vi "RSZVB Set Soft Key Label.vi"(8 "error in (no error)":errorcluster {"code" format="%.0x"}, 9 "Label":string, 10 "Key Number (1)":i32=1, 11 "VISA session":refnum<visa-resource-name>) -> (0 "error out":errorcluster {"code" format="%.0x"}, 3 "dup VISA session":refnum<visa-resource-name>)   [LabVIEW 2011]
doc: "This VI assigns the label to the soft key 1...8. The label may contain the '\\n'- character to form multiline labels.\n\nRemote-control command(s):\n:SYSTem:USER:FKEY 0\n:SYSTem:USER:FKEY <1...8>,'<Label>'"
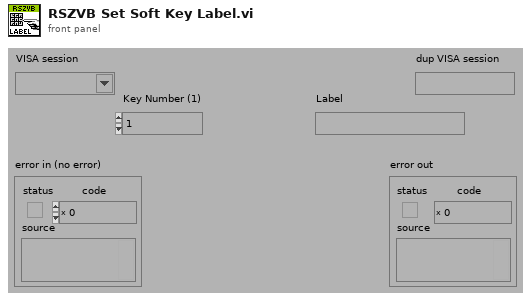
[diagram p1: front panel]
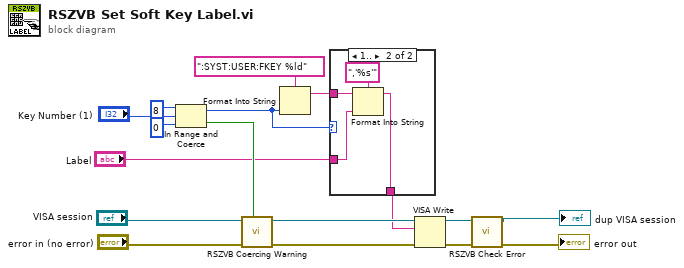
[diagram p0: block diagram]
diagram:
  n1 = In Range and Coerce(upper limit=8, x="Key Number (1)", lower limit=0) -> (coerced(x)=w6:i32, In Range?=w7:bool)
  n2 = call "RSZVB Coercing Warning.vi"("In Range?"=w7, "error in (no error)"="error in (no error)", "VISA session"="VISA session") -> ("error out"=w13:errorcluster, "dup VISA session"=w14:refnum<visa-resource-name>)  [unwired: 7 in]
  n3 = Format Into String(format string=":SYST:USER:FKEY %ld", w6) -> (resulting string=w5:string)  [unwired: 2 in, 1 out]
  n4 = case shown="1.." w6 {
    tunnel: w5 -> [w18 w20]
    tunnel: [w18 w19] -> w4
    tunnel: "Label" -> [_ w21]
    frame 0, Default {
    }
    frame 1.. {
      n5 = Format Into String(format string=",'%s'", initial string=w20, w21) -> (resulting string=w19:string)  [unwired: 1 in, 1 out]
    }
  }
  n6 = VISA Write(VISA resource name=w14, write buffer=w4, error in (no error)=w13) -> (VISA resource name out=w11:refnum<visa-resource-name>, error out=w12:errorcluster)  [unwired: 1 out]
  n7 = call "RSZVB Check Error.vi"("error in (no error)"=w12, "VISA session"=w11) -> ("error out"=→"error out":errorcluster, "dup VISA session"=→"dup VISA session":refnum<visa-resource-name>)  [unwired: 8 in]
